vi "Colonoscopy Competition_Differentiate_encoder.vi"(7 "Measurement Width (Counts)":i64=4, 9 "Encoder interval 2 (uS)":i64, 10 "Encoder interval 1 (uS)":i64) -> (2 "Enc 2 Vel. (Counts Per S)":dbl, 3 "Enc 1 Vel.(Counts perS)":dbl)   [LabVIEW 2016]
panel:
  # "INPUTS"
  # "OUTPUTS"
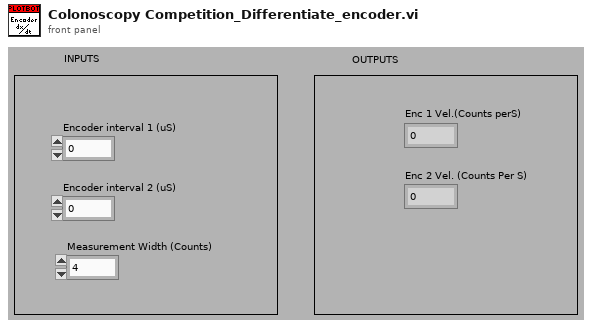
[diagram p1: front panel]
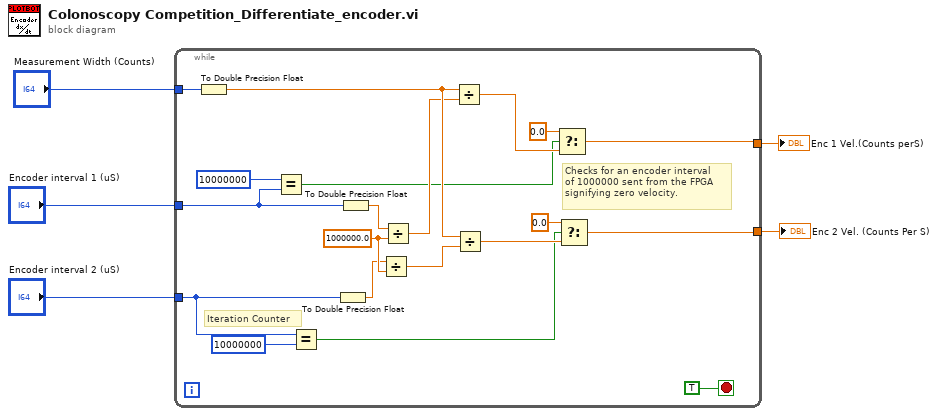
[diagram p0: block diagram]
diagram:
  n1 = while {
    tunnel: [w24] -> w5
    tunnel: [w23] -> w4
    tunnel: "Encoder interval 2 (uS)" -> [w7]
    tunnel: "Encoder interval 1 (uS)" -> [w11]
    tunnel: "Measurement Width (Counts)" -> [w12]
    stop <- TRUE stop-if-true
    w19 = 1000000.0 ("y")
    # "Checks for an encoder interval \nof 1000000 sent from the FPGA \nsignifying zero velocity."
    # "Iteration Counter"
    n2 = To Double Precision Float(number=w12) -> (double precision float=w20:dbl)
    n3 = Equal?(x=i64 10000000 ("t"), y=w11) -> (x = y?=w9:bool)
    n4 = Equal?(x=w7, y=i64 10000000 ("t")) -> (x = y?=w6:bool)
    n5 = To Double Precision Float(number=w7) -> (double precision float=w17:dbl)
    n6 = To Double Precision Float(number=w11) -> (double precision float=w18:dbl)
    n7 = Divide(x=w17, y=w19) -> (x/y=w15:dbl)
    n8 = Divide(x=w18, y=w19) -> (x/y=w16:dbl)
    n9 = Divide(x=w20, y=w16) -> (x/y=w14:dbl)
    n10 = Divide(x=w20, y=w15) -> (x/y=w13:dbl)
    n11 = Select(t=0.0, s=w9, f=w14) -> (s? t:f=w23:dbl)
    n12 = Select(t=0.0, s=w6, f=w13) -> (s? t:f=w24:dbl)
  }
  "Enc 2 Vel. (Counts Per S)" <- w5
  "Enc 1 Vel.(Counts perS)" <- w4
